vi "Math-Discrete Truncated Gaussian RNG.vi"(0 "samples":i32, 1 "reset":bool, 5 "Min":dbl, 7 "Max":dbl, 9 "Step":dbl, 11 "mu":dbl, 12 "sigma":dbl, 13 "seed":i32=-1) -> (4 "Array":dbl[](array[numeric]))   [LabVIEW 2020]
uses:
  LinSpace (start-stop-step).vi
  <vilib>/Analysis/NI_AALPro.lvlib
panel:
  out "Histogram":T1(graph)
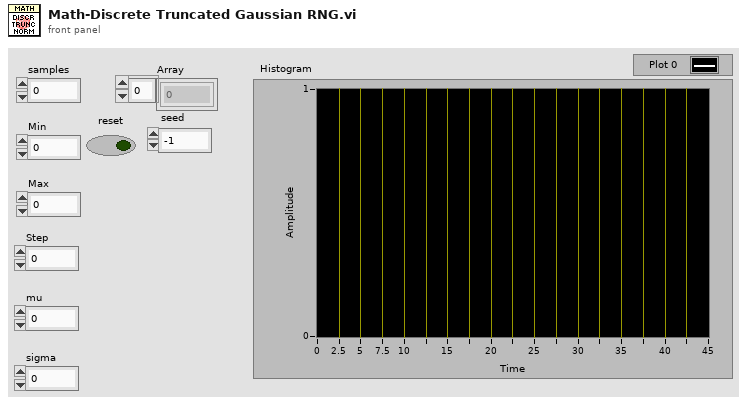
[diagram p1: front panel]
types:
  T1 = cluster{"X Values":dbl[], "Histogram: h(x)":i32[]}
  T2 = cluster{dbl, dbl, "inclusion":enum32{"lower", "upper"}}
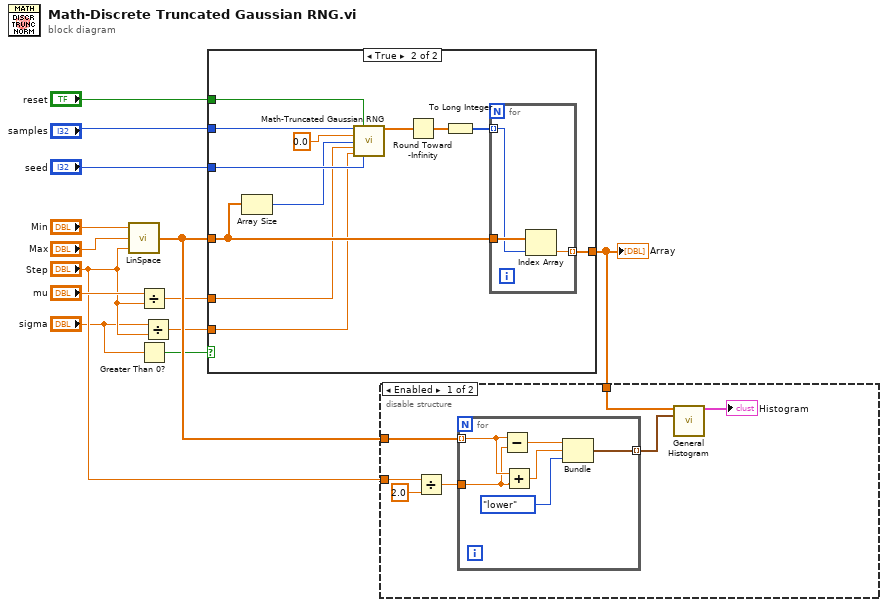
[diagram p0: block diagram]
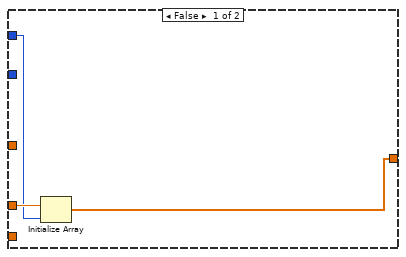
[diagram p2: hidden frame]
diagram:
  n1 = call-poly "LinSpace.vi"("Step"="Step", "Stop"="Max", "Start"="Min") -> ("Array"=w12:dbl[])  [unwired: 1 in, 1 out]
  n2 = Divide(x="mu", y="Step") -> (x/y=w3:dbl)
  n3 = Greater Than 0?(x="sigma") -> (x > 0?=w1:bool)
  n4 = Divide(x="sigma", y="Step") -> (x/y=w2:dbl)
  n5 = case shown="True" w1 {
    tunnel: [w14 w28] -> w13
    tunnel: w12 -> [_ w27]
    tunnel: "samples" -> [w15 w26]
    tunnel: "seed" -> [_ w25]
    tunnel: "reset" -> [_ w24]
    tunnel: w3 -> [w16 w19]
    tunnel: w2 -> [_ w18]
    frame False {
      n6 = Initialize Array(w16, w15) -> (w14:dbl[])
    }
    frame True {
      n7 = Array Size(array=w27) -> (size(s)=w21:i32)
      n8 = call "Math-Truncated Gaussian RNG.vi"("samples"=w26, "reset"=w24, "Min"=0.0, "Max"=w21, "mu"=w19, "sigma"=w18, "seed"=w25) -> ("Array"=w17:dbl[])  [unwired: 8 in]
      n9 = Round Toward -Infinity(1:w17) -> (0:w23:dbl[])
      n10 = To Long Integer(number=w23) -> (32bit integer=w22:i32[])
      n11 = for {
        tunnel: w22 -> [w30] mode=indexing
        tunnel: w27 -> [w31]
        tunnel: [w29] -> w28 mode=indexing
        n12 = Index Array(array=w31, index=w30) -> (element=w29:dbl)
      }
    }
  }
  "Array" <- w13
  n13 = disable-structure shown="Enabled" {
    disable-tunnel: w13 -> [w38 _]
    disable-tunnel: w12 -> [w37 _]
    disable-tunnel: "Step" -> [w33 _]
    frame Enabled {
      n14 = Divide(x=w33, y=2.0) -> (x/y=w35:dbl)
      n15 = for {
        tunnel: w37 -> [w44] mode=indexing
        tunnel: w35 -> [w43]
        tunnel: [w39] -> w34 mode=indexing
        n16 = Subtract(x=w44, y=w43) -> (x-y=w42:dbl)
        n17 = Add(x=w44, y=w43) -> (x+y=w41:dbl)
        n18 = Bundle(w42, w41, "inclusion"=enum32{"lower", "upper"}."lower") -> (w39:T2)  [unwired: 1 in]
      }
      n19 = call <vilib>:"General Histogram.vi"("X"=w38, "Bins"=w34) -> ("Histogram Graph"=→"Histogram":T1)  [unwired: 9 in, 4 out]
    }
    frame Disabled {
    }
  }
